vi "GetType.vi"(8 "error in (no error)":errorcluster, 11 "Configure Acquisition Record Msg in":refnum<class "Configure Acquisition Record Msg.lvclass">) -> (0 "error out":errorcluster, 2 "Data Sample":variant, 3 "Configure Acquisition Record Msg out":refnum<class "Configure Acquisition Record Msg.lvclass">)   [LabVIEW 2014, in "CS++Scope.lvlib" / "Configure Acquisition Record Msg.lvclass"]
doc: "This VI delivers a sample of the data type format the message expects."
uses:
  Configure Acquisition Record Msg.lvclass
  Configure Acquisition Record Msg.lvclass/Configure Acquisition Record Msg.ctl
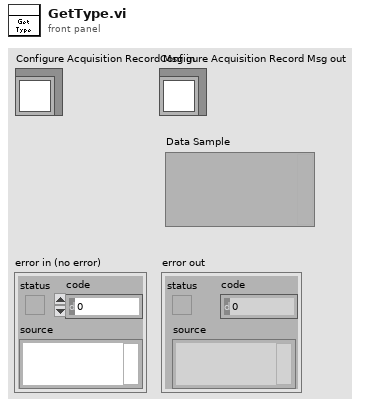
[diagram p1: front panel]
types:
  T1 = cluster{"time per record (1.0E-3 s)":dbl[unit], "min record length (100 samples)":i32, "acquisition start time (0.0 s)":dbl[unit]}
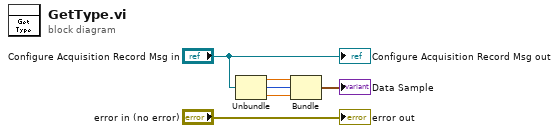
[diagram p0: block diagram]
diagram:
  n1 = Unbundle("Configure Acquisition Record Msg in") -> (w4:dbl[unit], w3:i32, w2:dbl[unit])
  n2 = Bundle("time per record (1.0E-3 s)"=w4, "min record length (100 samples)"=w3, "acquisition start time (0.0 s)"=w2) -> (→"Data Sample":T1)  [unwired: 1 in]
  "error out" <- "error in (no error)"
  "Configure Acquisition Record Msg out" <- "Configure Acquisition Record Msg in"
